vi "Convert Temperature.vi"(7 "1-Wire DIO Pin":refnum<k21>="ConnectorA/DIO15", 8 "error in (no error)":errorcluster, 11 "Powered Device? (T)":bool=TRUE) -> (0 "error out":errorcluster, 2 "Convert Time (usec)":u32)   [LabVIEW 2014, in "Maxim 1-Wire.lvlib"]
doc: "SEARCH ROM [F0h]\nWhen a system is initially powered up, the master must identify the ROM codes of all slave devices on the bus, which allows the master to determine the number of slaves and their device types. The master learns the ROM codes through a process of elimination that requires the master to perform a Search ROM cycle (i.e., Search ROM command followed by data exchange) as many times as necessary to identify all of the slave devices. If there is only one slave on the bus, the simpler Read ROM command (see below) can be used in place of the Search ROM process. For a detailed explanation of the Search ROM procedure, refer to the iButton® Book of Standards at www.maxim-ic.com/ibuttonbook. After every Search ROM cycle, the bus master must return to Step 1 (Initialization) in the transaction sequence."
uses:
  Maxim 1-Wire.lvlib
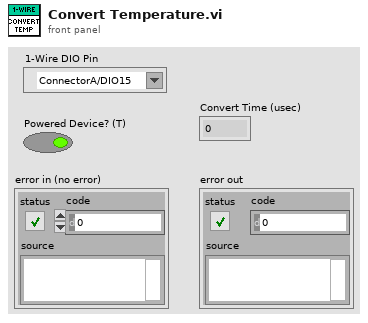
[diagram p1: front panel]
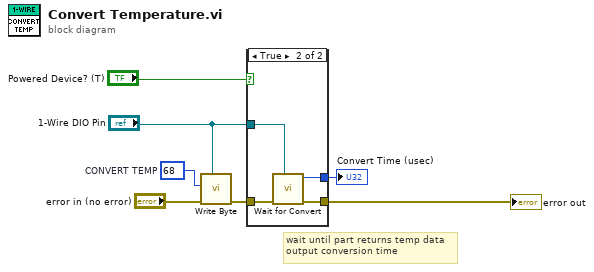
[diagram p0: block diagram]
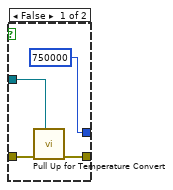
[diagram p2: hidden frame]
diagram:
  w7 = u8 68  # CONVERT TEMP
  # "wait until part returns temp data\noutput conversion time"
  n1 = call "Write Byte.vi"("1-Wire DIO Pin"="1-Wire DIO Pin", "error in"="error in (no error)", "Tx data"=w7) -> ("error out"=w5:errorcluster)  [unwired: 8 in]
  n2 = case shown="True" "Powered Device? (T)" {
    tunnel: [w10 w15] -> w6
    tunnel: w5 -> [w11 w14]
    tunnel: "1-Wire DIO Pin" -> [w9 w13]
    tunnel: [u32 750000 ("Convert Time (usec)") w12] -> w2
    frame False {
      n3 = call "Pull Up for Temperature Convert.vi"("1-Wire DIO Pin"=w9, "error in"=w11) -> ("error out"=w10:errorcluster)  [unwired: 9 in]
    }
    frame True {
      n4 = call "Wait for Convert.vi"("1-Wire DIO Pin"=w13, "error in"=w14) -> ("error out"=w15:errorcluster, "Convert Time (usec)"=w12:u32)  [unwired: 8 in]
    }
  }
  "error out" <- w6
  "Convert Time (usec)" <- w2
